vi "Create Connection.vi"(8 "error in (no error)":errorcluster, 11 "TCP Client in":refnum<class "TCP Client.lvclass">) -> (0 "error out":errorcluster, 2 "Connection":refnum<class "IConnection.lvclass">, 3 "TCP Client out":refnum<class "TCP Client.lvclass">)   [LabVIEW 2019, in "TCP Client.lvclass"]
uses:
  <vilib>/gpm_packages/@cs/Network-interface/Source/TCP Interface/TCP Client/TCP Client.lvclass
  <vilib>/gpm_packages/@cs/Network-interface/Source/Connection Reference/IConnection/IConnection.lvclass
  <vilib>/gpm_packages/@cs/Network-interface/Source/TCP Interface/TCP Client/TCP Client.lvclass/TCP Client.ctl
  <vilib>/gpm_packages/@cs/Network-interface/Source/TCP Interface/TCP Connection/TCP Connection.lvclass
  C:/Program Files/National Instruments/LabVIEW 2019/vi.lib/gpm_packages/@cs/Network-interface/Source/Connection Reference/IConnection/IConnection.lvclass
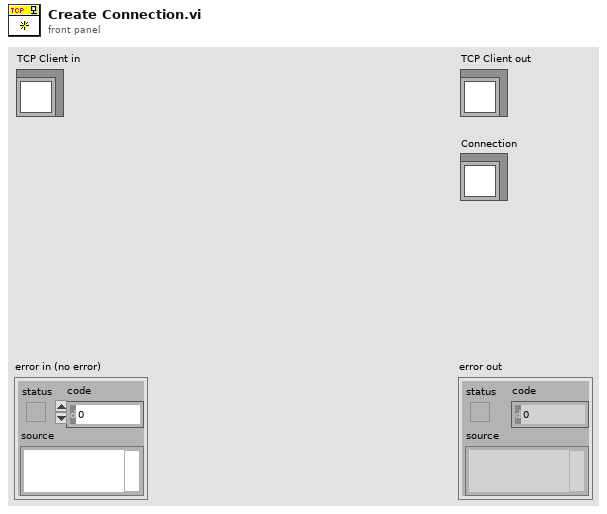
[diagram p1: front panel]
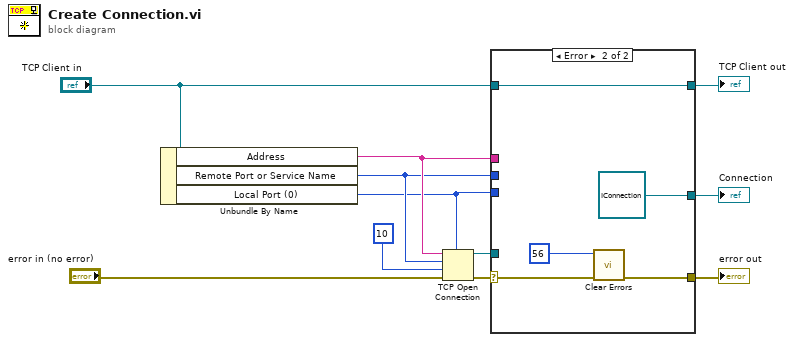
[diagram p0: block diagram]
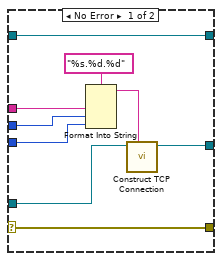
[diagram p2: hidden frame]
diagram:
  n1 = Unbundle By Name("TCP Client in") -> ("Address"=w3:string, "Remote Port or Service Name"=w2:u16, "Local Port (0)"=w1:u16)
  n2 = TCP Open Connection(address=w3, remote port or service name=w2, timeout ms (60000)=10 ("Timeout (25000 ms)"), local port=w1, error in (no error)="error in (no error)") -> (connection ID=w8:refnum<k5>, error out=w9:errorcluster)
  n3 = case shown="Error" w9 {
    selector: w9 -> [w17 w24]
    tunnel: w8 -> [w19 _]
    tunnel: "TCP Client in" -> [w20 w25]
    tunnel: [w20 w25] -> w6
    tunnel: [w18 refnum<class "IConnection.lvclass"> refnum ("Connection")] -> w5
    tunnel: [w17 w22] -> w4
    tunnel: w3 -> [w12 _]
    tunnel: w2 -> [w14 _]
    tunnel: w1 -> [w13 _]
    frame No Error {
      n4 = Format Into String(format string="%s.%d.%d", w12, w14, w13) -> (resulting string=w16:string)  [unwired: 2 in, 1 out]
      n5 = call <vilib>:"Construct TCP Connection.vi"("ID"=w16, "ConnectionRef"=w19) -> ("TCP Connection out"=w18:refnum<class "TCP Connection.lvclass">)  [unwired: 9 in]
    }
    frame Error {
      n6 = call <vilib>:"Clear Errors.vi"("error in (no error)"=w24, "specific error code to clear (0: all)"=56) -> ("error out"=w22:errorcluster)  [unwired: 4 in, 1 out]
    }
  }
  "error out" <- w4
  "TCP Client out" <- w6
  "Connection" <- w5
